vi "Config case parse cmd.vi"(10 "Msg in":T1, 11 "Seperator":string[](array[string])) -> (2 "Parsed CMD":T2, 3 "Command":string)   [LabVIEW 2020]
uses:
  parsed device cmd.ctl
  BaseDriver/DriverMsg.ctl
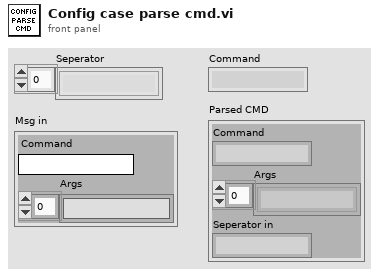
[diagram p1: front panel]
types:
  T1 = typedef "DriverMsg.ctl" = cluster{"Command":string, "Args":string[]}
  T2 = typedef "parsed device cmd.ctl" = cluster{"Command":string, "Args":string[], "Seperator in":string}
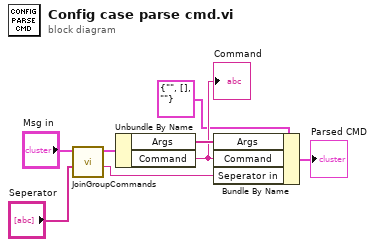
[diagram p0: block diagram]
diagram:
  n1 = call "JoinGroupCommands.vi"("Seperator between var name and chan num"="Seperator", "Msg in"="Msg in") -> ("Seperator out"=w7:string, "Msg out"=w2:T1)  [unwired: 6 in, 2 out]
  n2 = Unbundle By Name(w2) -> ("Args"=w6:string[], "Command"=w5:string)
  "Command" <- w5
  n3 = Bundle By Name(cluster=T2 {"Command"="", "Args"=[], "Seperator in"=""} ("Parsed CMD"), "Args"=w6, "Command"=w5, "Seperator in"=w7) -> (→"Parsed CMD":T2)
